vi "LP_Butter.vi"(1 "High cutoff freq":dbl=0.45000000000000007 format="%0.2f", 2 "Samping Frequency":dbl, 3 "Signal Sequence":dbl[](array[numeric])) -> (0 "reversed array":dbl[](array[numeric]))   [LabVIEW 2019]
uses:
  <vilib>/Analysis/3filter.llb/Filter Passband Type.ctl
  <vilib>/Analysis/3filter.llb/Butterworth Filter (DBL).vi
  <vilib>/Analysis/NI_AALBase.lvlib
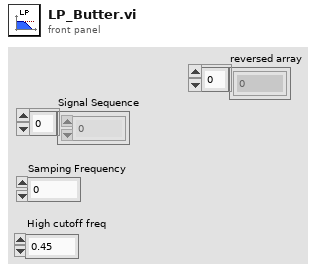
[diagram p1: front panel]
types:
  T1 = typedef "NI_AALBase.lvlib/Filter Passband Type.ctl" = enum32{"Lowpass", "Highpass", "Bandpass", "Bandstop"}
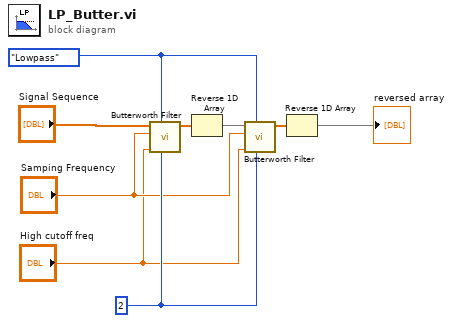
[diagram p0: block diagram]
diagram:
  w3 = Filter_Passband_Type."Lowpass" ("filter type")
  w8 = 2 ("order")
  n1 = call-poly <vilib>:"Butterworth Filter.vi"("order"=w8, "filter type"=w3, "low cutoff freq: fl"="High cutoff freq", "sampling freq: fs"="Samping Frequency", "X"="Signal Sequence") -> ("Filtered X"=w4:dbl[])  [unwired: 3 in, 1 out]
  n2 = Reverse 1D Array(array=w4) -> (reversed array=w5:dbl[])
  n3 = call-poly <vilib>:"Butterworth Filter.vi"("order"=w8, "filter type"=w3, "low cutoff freq: fl"="High cutoff freq", "sampling freq: fs"="Samping Frequency", "X"=w5) -> ("Filtered X"=w6:dbl[])  [unwired: 3 in, 1 out]
  n4 = Reverse 1D Array(array=w6) -> (reversed array=→"reversed array":dbl[])
